vi "Main.vi"() -> ()   [LabVIEW 2011]
panel:
  in  "Три":bool
  out "String":string="Один"
  in  "stop":bool
  in  "Два":bool
  in  "Один":bool
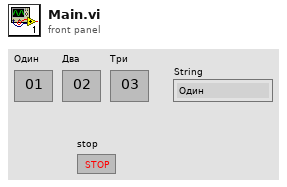
[diagram p1: front panel]
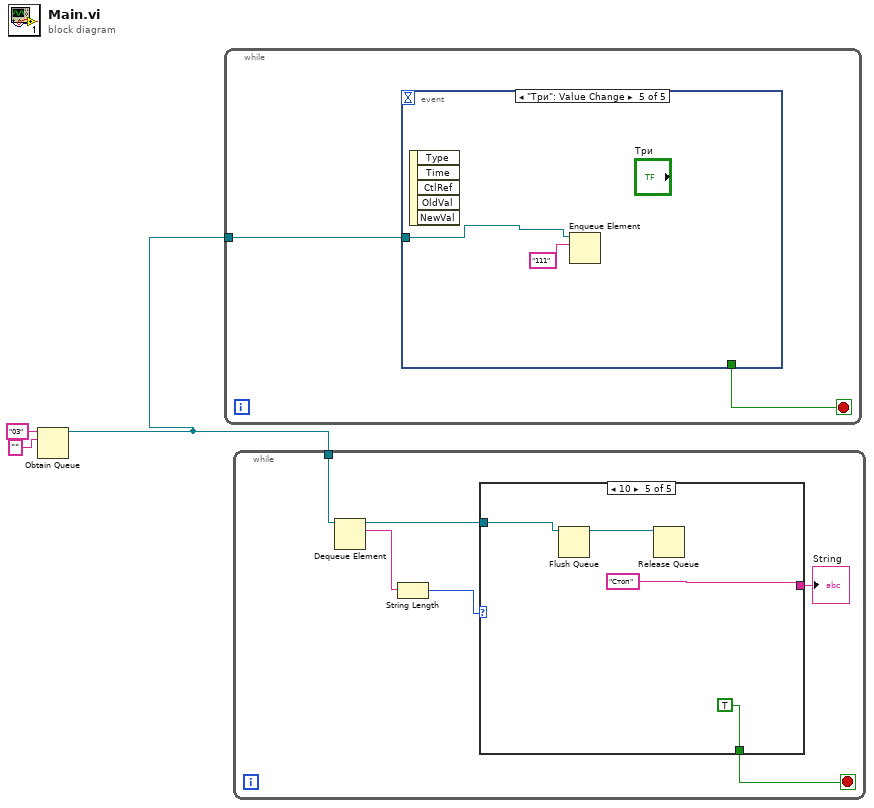
[diagram p0: block diagram]
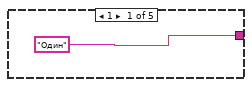
[diagram p2: hidden frame]
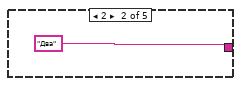
[diagram p3: hidden frame]
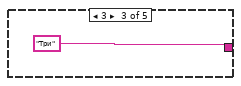
[diagram p4: hidden frame]
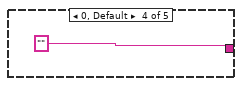
[diagram p5: hidden frame]
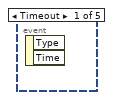
[diagram p6: hidden frame]
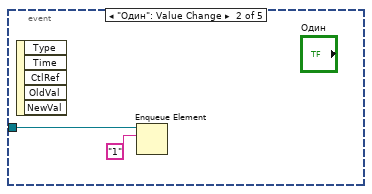
[diagram p7: hidden frame]
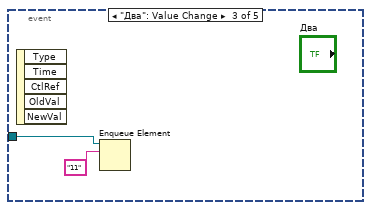
[diagram p8: hidden frame]
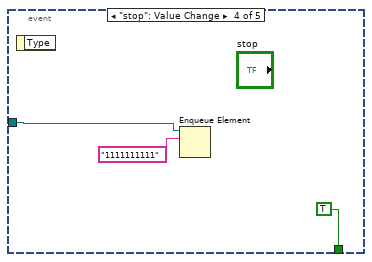
[diagram p9: hidden frame]
diagram:
  n1 = Obtain Queue(name (unnamed)="03", element data type="" ("name (unnamed)")) -> (queue out=w1:refnum<queue>)  [unwired: 3 in, 2 out]
  n2 = while {
    tunnel: w1 -> [w5]
    stop <- w4 stop-if-true
    n3 = event shown="[4] \"Три\": Value Change" {
      selector: _ -> [_ _ _ _ _]
      dyn-events: _ -> [_ _ _ _ _]
      timeout: _ -> [_ _ _ _ _]
      tunnel: w5 -> [_ w7 w8 w11 w13]
      tunnel: [_ _ _ TRUE _] -> w4
      event Timeout {
        n4 = event-data() -> ()  [unwired: 1 in, 2 out]
      }
      event "Один": Value Change {
        n5 = event-data() -> ()  [unwired: 1 in, 5 out]
        n6 = Enqueue Element(queue=w7, element="1") -> ()  [unwired: 2 in, 3 out]
      }
      event "Два": Value Change {
        n7 = event-data() -> ()  [unwired: 1 in, 5 out]
        n8 = Enqueue Element(queue=w8, element="11") -> ()  [unwired: 2 in, 3 out]
      }
      event "stop": Value Change {
        n9 = event-data() -> ()  [unwired: 1 in, 1 out]
        n10 = Enqueue Element(queue=w11, element="1111111111") -> ()  [unwired: 2 in, 3 out]
      }
      event "Три": Value Change {
        n11 = event-data() -> ()  [unwired: 1 in, 5 out]
        n12 = Enqueue Element(queue=w13, element="111") -> ()  [unwired: 2 in, 3 out]
      }
    }
  }
  n13 = while {
    tunnel: w1 -> [w20]
    stop <- w16 stop-if-true
    n14 = Dequeue Element(queue=w20) -> (queue out=w15:refnum<queue>, element=w19:string)  [unwired: 2 in, 2 out]
    n15 = String Length(string=w19) -> (length=w18:i32)
    n16 = case shown="10" w18 {
      tunnel: ["Один" "Два" "Три" "" "Стоп"] -> w17
      tunnel: [_ _ _ _ TRUE] -> w16
      tunnel: w15 -> [_ _ _ _ w26]
      frame 1 {
      }
      frame 2 {
      }
      frame 3 {
      }
      frame 0, Default {
      }
      frame 10 {
        n17 = Flush Queue(queue=w26) -> (queue out=w25:refnum<queue>)  [unwired: 1 in, 2 out]
        n18 = Release Queue(queue=w25) -> ()  [unwired: 2 in, 3 out]
      }
    }
    "String" <- w17
  }
